vi "计算第一个点在影像坐标系的理论位置.vi"(9 "第一个点与参考点在产品坐标系位置差":cluster{"X":sgl, "Y":sgl}={"X"=-237.0, "Y"=135.0}, 10 "参考点影像坐标":cluster{"X":sgl, "Y":sgl}, 11 "Angle (Pixel)":dbl) -> (3 "第一个点在影像坐标系坐标":cluster{dbl, dbl})   [LabVIEW 2014]
uses:
  <vilib>/Analysis/coordinate.llb/2D Cartesian Coordinate Rotation (Scalar).vi
  <vilib>/Analysis/NI_AALPro.lvlib
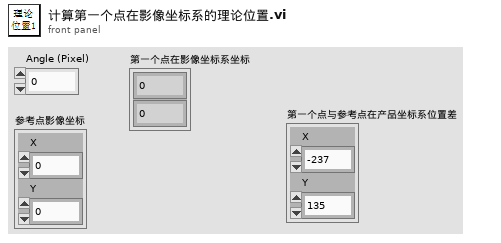
[diagram p1: front panel]
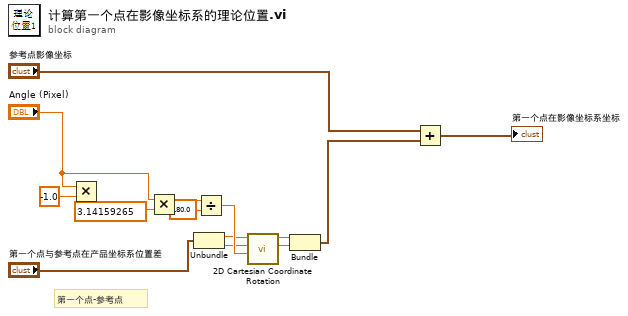
[diagram p0: block diagram]
diagram:
  # "第一个点-参考点"
  n1 = Multiply(x="Angle (Pixel)", y=-1.0) -> ()  [unwired: 1 out]
  n2 = Multiply(x="Angle (Pixel)", y=3.14159265) -> (x*y=w12:dbl)
  n3 = Unbundle("第一个点与参考点在产品坐标系位置差") -> ("X"=w2:sgl, "Y"=w3:sgl)
  n4 = Divide(x=w12, y=180.0) -> (x/y=w14:dbl)
  n5 = call-poly <vilib>:"2D Cartesian Coordinate Rotation.vi"("theta"=w14, "y"=w3, "x"=w2) -> ("y out"=w5:dbl, "x out"=w4:dbl)  [unwired: 6 in, 1 out]
  n6 = Bundle("x out"=w4, "y out"=w5) -> (w8:cluster{"x out":dbl, "y out":dbl})  [unwired: 1 in]
  n7 = Add(x="参考点影像坐标", y=w8) -> (x+y=→"第一个点在影像坐标系坐标":cluster{dbl, dbl})
